vi "asset.search.vi"(5 "property value":string, 7 "property key":string, 8 "error in":errorcluster, 9 "label":string, 10 "search text":string, 11 "Client in":refnum<class "Client.lvclass">) -> (0 "error out":errorcluster, 2 "List":refnum<class "List.lvclass">, 3 "Client out":refnum<class "Client.lvclass">)   [LabVIEW 2020, in "Client.lvclass"]
doc: "Searches for assets matching the given text, label, and/or property filters and returns a handle list of matches."
uses:
  Client.lvclass
  List/List.lvclass
  Client.lvclass/Client.ctl
  List/List.lvclass/List.ctl
  client.lvlib
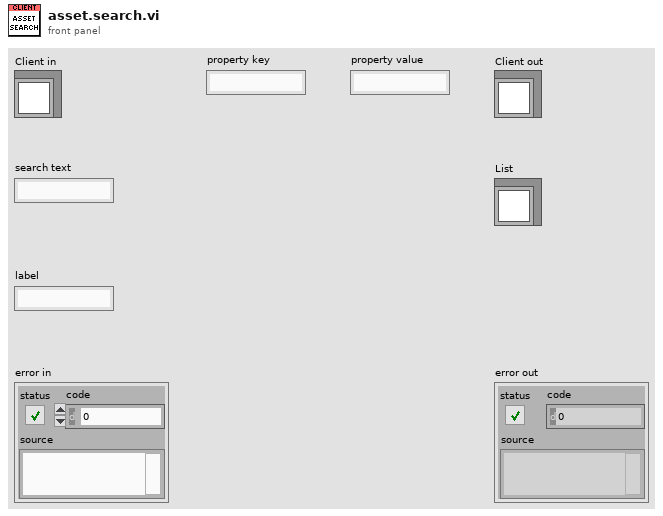
[diagram p1: front panel]
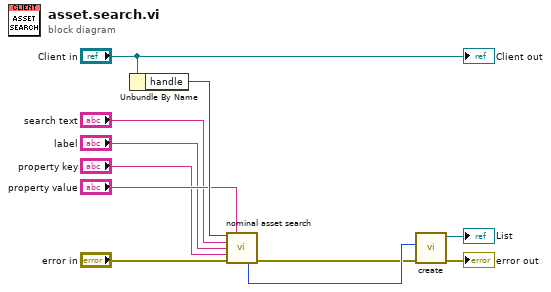
[diagram p0: block diagram]
diagram:
  n1 = Unbundle By Name("Client in") -> ("handle"=w10:i32)
  n2 = call "nominal asset search.vi"("client"=w10, "property_value"="property value", "search_text"="search text", "label"="label", "property_key"="property key", "error in (no error)"="error in") -> ("out_list out"=w4:i32, "error out"=w3:errorcluster)  [unwired: 6 in, 2 out]
  n3 = call "create.vi"("error in (no error)"=w3, "handle"=w4) -> ("error out"=→"error out":errorcluster, "List out"=→"List":refnum<class "List.lvclass">)  [unwired: 8 in]
  "Client out" <- "Client in"
